vi "rx_response.vi"(8 "error in":errorcluster, 11 "msg in":string="A\u0002F\u0001\u0000\u0000E\u0002") -> (0 "error out":errorcluster, 1 "rx msg":T1={"cmd"="F", "payload"="", "cs"=""}, 2 "msg complete":bool, 3 "remain":string)   [LabVIEW 2019]
uses:
  type_rxmsg.ctl
panel:
  out "payload length":u16
  out "after start":string
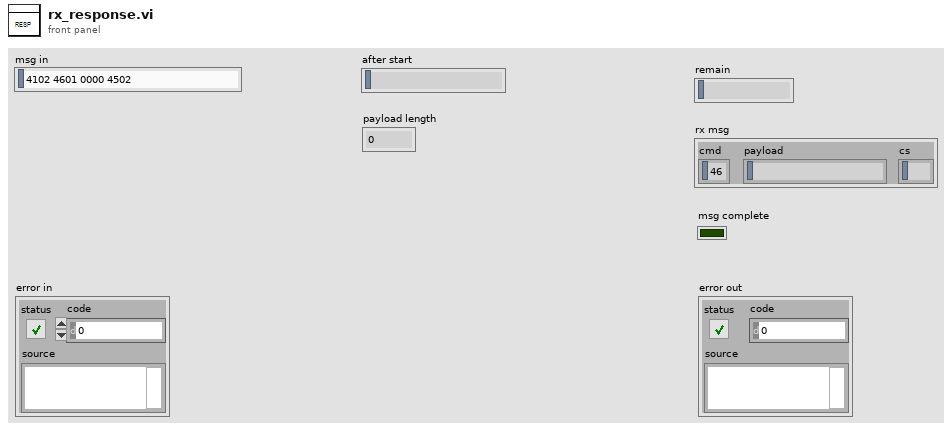
[diagram p1: front panel]
types:
  T1 = typedef "type_rxmsg.ctl" = cluster{"cmd":string, "payload":string, "cs":string}
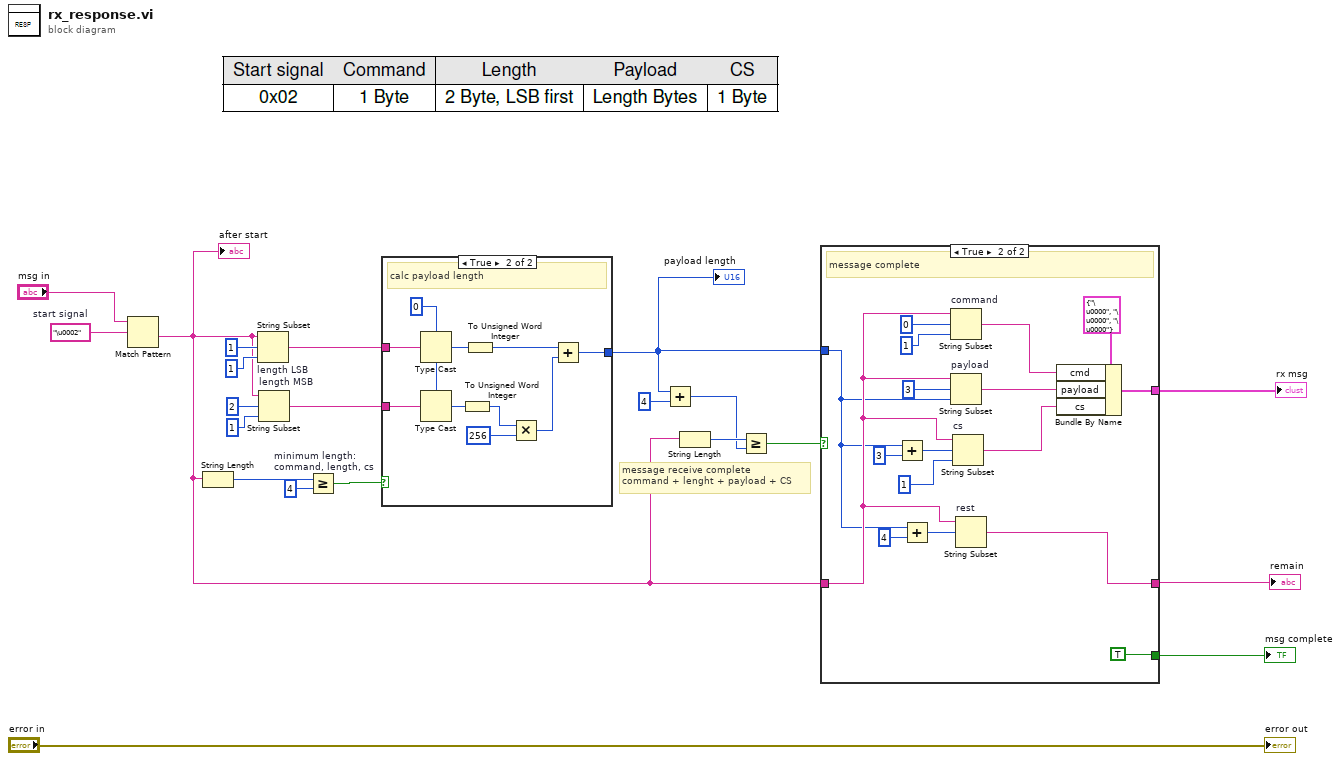
[diagram p0: block diagram]
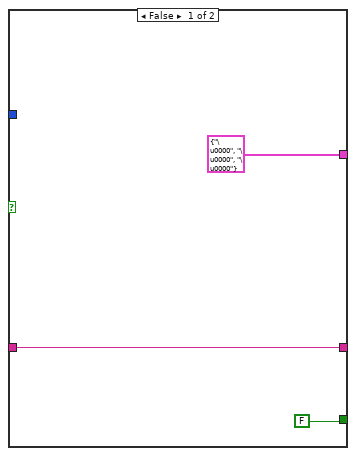
[diagram p2: hidden frame]
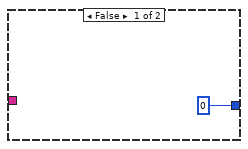
[diagram p3: hidden frame]
diagram:
  w21 = "\u0002"  # start signal
  # "message receive complete\ncommand + lenght + payload + CS"
  n1 = Match Pattern(string="msg in", regular expression=w21) -> (after substring=w8:string)  [unwired: 1 in, 3 out]
  "after start" <- w8
  n2 = String Length(string=w8) -> (length=w20:i32)
  n3 = String Subset "length LSB"(string=w8, offset (0)=1, length (rest)=1 ("length (rest)")) -> (substring=w13:string)
  n4 = String Subset "length MSB"(string=w8, offset (0)=2, length (rest)=1 ("length (rest)")) -> (substring=w12:string)
  n5 = Greater Or Equal? "minimum length:\ncommand, length, cs"(x=w20, y=4) -> (x >= y?=w18:bool)
  n6 = case shown="True" w18 {
    tunnel: w13 -> [_ w32]
    tunnel: w12 -> [_ w31]
    tunnel: [u16 0 w23] -> w4
    frame False {
    }
    frame True {
      w30 = u8 0 ("CMD_SCANSTART_REQ")
      # "calc payload length"
      n7 = Type Cast(type=w30, x=w32) -> (*(type *) &x=w26:u8)
      n8 = Type Cast(type=w30, x=w31) -> (*(type *) &x=w27:u8)
      n9 = To Unsigned Word Integer(number=w27) -> (unsigned 16bit integer=w28:u16)
      n10 = To Unsigned Word Integer(number=w26) -> (unsigned 16bit integer=w24:u16)
      n11 = Multiply(x=w28, y=u16 256) -> (x*y=w25:u16)
      n12 = Add(x=w24, y=w25) -> (x+y=w23:u16)
    }
  }
  "payload length" <- w4
  n13 = Add(x=w4, y=u16 4) -> (x+y=w5:u16)
  n14 = String Length(string=w8) -> (length=w11:i32)
  n15 = Greater Or Equal?(x=w11, y=w5) -> (x >= y?=w9:bool)
  n16 = case shown="True" w9 {
    tunnel: w8 -> [w35 w44]
    tunnel: [w35 w43] -> w6
    tunnel: w4 -> [_ w42]
    tunnel: [T1 {"cmd"="\u0000", "payload"="\u0000", "cs"="\u0000"} ("rx msg") w37] -> w3
    tunnel: [FALSE TRUE] -> w2
    frame False {
    }
    frame True {
      # "message complete"
      n17 = Add(x=w42, y=u16 3) -> (x+y=w49:u16)
      n18 = Add(x=w42, y=u16 4) -> (x+y=w45:u16)
      n19 = String Subset "command"(string=w44, offset (0)=0, length (rest)=1 ("length (rest)")) -> (substring=w39:string)
      n20 = String Subset "payload"(string=w44, offset (0)=3, length (rest)=w42) -> (substring=w40:string)
      n21 = String Subset "cs"(string=w44, offset (0)=w49, length (rest)=1 ("length (rest)")) -> (substring=w38:string)
      n22 = String Subset "rest"(string=w44, offset (0)=w45) -> (substring=w43:string)  [unwired: 1 in]
      n23 = Bundle By Name(cluster=T1 {"cmd"="\u0000", "payload"="\u0000", "cs"="\u0000"} ("rx msg"), "cmd"=w39, "payload"=w40, "cs"=w38) -> (w37:T1)
    }
  }
  "remain" <- w6
  "rx msg" <- w3
  "msg complete" <- w2
  "error out" <- "error in"
